vi "SbigReadOut.vi"(0 "error in (no error)":errorcluster, 2 "Sbig":T1, 5 "CCD":u16(ring) items=["IMAGING", "TRACKING"], 6 "Binning Mode":u16(ring) items=["1x1", "2x2", "3x3"], 7 "Window":T2) -> (3 "error out":errorcluster, 8 "Image":i32[][](graph))   [LabVIEW 2009]
uses:
  Controls/SbigReference.ctl
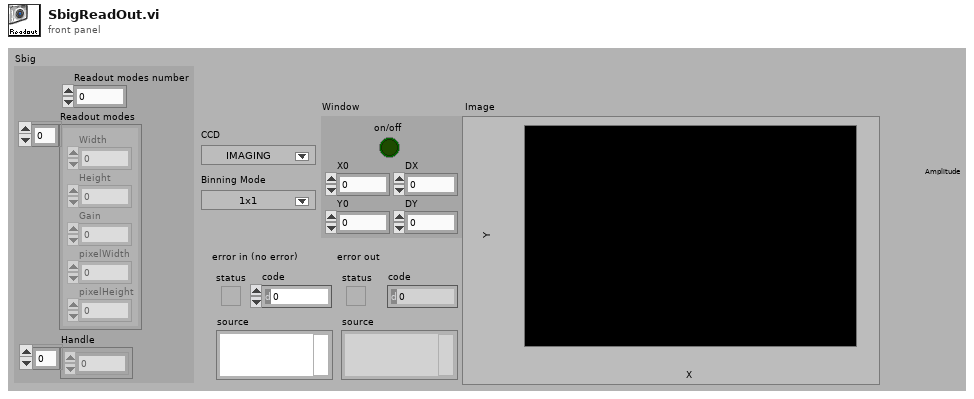
[diagram p1: front panel]
types:
  T1 = typedef "SbigReference.ctl" = cluster{"Readout modes number":u16, "Readout modes":cluster{"Width":u16, "Height":u16, "Gain":dbl, "pixelWidth":dbl, "pixelHeight":dbl}[], "Handle":u16[]}
  T2 = cluster{"X0":u16, "Y0":u16, "DX":u16, "DY":u16, "on/off":bool}
  T3 = enum16{"0-NoCommand", "1-StartExposure", "2-EndExposure", "3-ReadoutLine", "4-DumpLines", "5-SetTemperatureRegulation", "6-QueryTemperatureStatus", "7-ActivateRelay", "8-PulseOut", "9-EstablishLink", "10-GetDriverInfo", "11-GetCCDInfo", "12-QueryCommandStatus", "13-MiscellaneousControl", "14-ReadSubstractLine", "15-UpdateClock", "16-ReadOffset", "17-OpenDriver", "18-CloseDriver", "19-TXSerialBytes", "20-GetSerialStatus", "21-AOTipTilt", "22-AOSetFocus", "23-AODelay", "24-GetTurboStatus", "25-EndReadout", "26-GetUSTimer", "27-OpenDevice", "28-CloseDevice", "29-SetIRQL", "30-GetIRQL", "31-GetLine", "32-GetLinkStatus", "33-GetDriverHandle", "34-SetDriverHandle", "35-StartReadout", "36-GetErrorString", "37-SetDriverControl", "38-GetDriverControl", "39-USBADControl", "40-QueryUSB", "41-GetPentiumCycleCount", "42-RWUSBI2C", "43-CFW"}
  T4 = cluster{"Width":u16, "Height":u16, "Gain":dbl, "pixelWidth":dbl, "pixelHeight":dbl}[]
  T5 = cluster{"Width":u16, "Height":u16, "Gain":dbl, "pixelWidth":dbl, "pixelHeight":dbl}
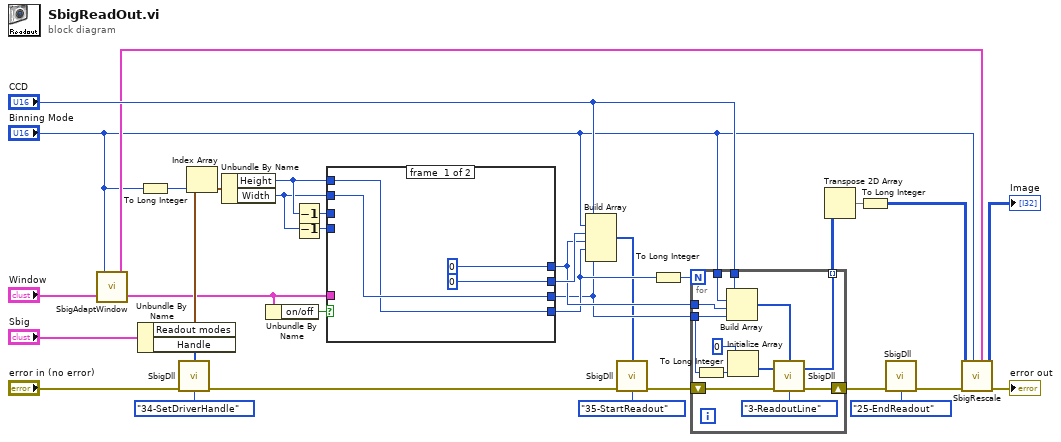
[diagram p0: block diagram]
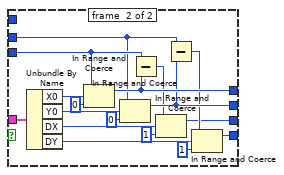
[diagram p2: hidden frame]
diagram:
  n1 = call "SbigAdaptWindow.vi"("Window in"="Window", "Binning Mode"="Binning Mode") -> ("Window out"=w8:T2, "Window out 2"=w5:T2)
  n2 = Unbundle By Name("Sbig") -> ("Readout modes"=w34:T4, "Handle"=w12:u16[])
  n3 = To Long Integer(number="Binning Mode") -> (32bit integer=w22:i32)
  n4 = call "SbigDll.vi"("error in (no error)"="error in (no error)", "Command"=T3."34-SetDriverHandle", "Parameters"=w12) -> ("error out"=w15:errorcluster)  [unwired: 1 in, 3 out]
  n5 = Index Array(array=w34, index=w22) -> (element=w32:T5)
  n6 = Unbundle By Name(w32) -> ("Height"=w29:u16, "Width"=w28:u16)
  n7 = Unbundle By Name(w8) -> ("on/off"=w33:bool)
  n8 = Decrement(x=w29) -> (x-1=w30:u16)
  n9 = Decrement(x=w28) -> (x-1=w31:u16)
  n10 = case shown="True" w33 {
    tunnel: w8 -> [_ w55]
    tunnel: [u16 0 ("X0") w50] -> w24
    tunnel: [u16 0 ("Y0") w49] -> w27
    tunnel: [w36 w40] -> w20
    tunnel: [w35 w39] -> w21
    tunnel: w29 -> [w35 _]
    tunnel: w28 -> [w36 _]
    tunnel: w31 -> [_ w48]
    tunnel: w30 -> [_ w47]
    frame #0 {
    }
    frame #1 {
      n11 = Unbundle By Name(w55) -> ("X0"=w54:u16, "Y0"=w52:u16, "DX"=w46:u16, "DY"=w45:u16)
      n12 = In Range and Coerce(upper limit=w48, x=w54, lower limit=u16 0 ("limite basse")) -> (coerced(x)=w50:u16)  [unwired: 1 out]
      n13 = In Range and Coerce(upper limit=w47, x=w52, lower limit=u16 0 ("limite basse")) -> (coerced(x)=w49:u16)  [unwired: 1 out]
      n14 = Subtract(x=w48, y=w50) -> (x-y=w42:u16)
      n15 = In Range and Coerce(upper limit=w42, x=w46, lower limit=u16 1 ("limite basse")) -> (coerced(x)=w40:u16)  [unwired: 1 out]
      n16 = Subtract(x=w47, y=w49) -> (x-y=w41:u16)
      n17 = In Range and Coerce(upper limit=w41, x=w45, lower limit=u16 1 ("limite basse")) -> (coerced(x)=w39:u16)  [unwired: 1 out]
    }
  }
  n18 = Build Array("CCD", "Binning Mode", w27, w24, w21, w20) -> (w16:u16[])
  n19 = call "SbigDll.vi"("error in (no error)"=w15, "Command"=T3."35-StartReadout", "Parameters"=w16) -> ("error out"=w17:errorcluster)  [unwired: 1 in, 3 out]
  n20 = To Long Integer(number=w21) -> (32bit integer=w26:i32)
  n21 = for {
    N: w26 -> [_]
    tunnel: "CCD" -> [w67]
    tunnel: "Binning Mode" -> [w66]
    tunnel: w24 -> [w65]
    tunnel: w20 -> [w60]
    tunnel: [w63] -> w19 mode=indexing
    shift-right: [w61] -> w23
    shift-left: w17 -> [w62]
    n22 = To Long Integer(number=w60) -> (32bit integer=w59:i32)
    n23 = Build Array(w67, w66, w65, w60) -> (w64:u16[])
    n24 = Initialize Array(u16 0 ("Nouvel élément"), w59) -> (w57:u16[])
    n25 = call "SbigDll.vi"("error in (no error)"=w62, "Command"=T3."3-ReadoutLine", "Results In"=w57, "Parameters"=w64) -> ("error out"=w61:errorcluster, "Results Out"=w63:u16[])  [unwired: 2 out]
  }
  n26 = Transpose 2D Array(2D array=w19) -> (transposed array=w18:u16[][])
  n27 = To Long Integer(number=w18) -> (32bit integer=w3:i32[][])
  n28 = call "SbigDll.vi"("error in (no error)"=w23, "Command"=T3."25-EndReadout") -> ("error out"=w7:errorcluster)  [unwired: 2 in, 3 out]
  n29 = call "SbigRescale.vi"("Window"=w5, "Binning Mode"="Binning Mode", "Image In"=w3, "error out 2"=w7) -> ("Image Out"=→"Image":i32[][], "error out"=→"error out":errorcluster)  [unwired: 3 out]
